vi "Shooter_Begin.vi"   [LabVIEW 2012]
uses:
  <vilib>/Rock Robotics/WPI/CAN/Jaguar/SubVIs/WPI_CANJaguar_ControlMode.ctl
  <vilib>/Rock Robotics/SystemInterfaces/DIO/FPGA_DIOChannel.ctl
  <vilib>/Rock Robotics/SystemInterfaces/Typedef/FPGA_TypedefDigitalModule.ctl
  <vilib>/Rock Robotics/WPI/CAN/Jaguar/SubVIs/WPI_CANJaguar_BrakeCoastMode.ctl
  Program Files (x86)/National Instruments/LabVIEW 2012/examples/FRC/I2C/ADXL345 I2C/Driver/ADXL345 I2C Range.ctl
  <vilib>/Rock Robotics/WPI/MotorControl/WPI_MotorControlOpenCANJaguar.vi
types:
  T1 = typedef "WPI_CANJaguar_BrakeCoastMode.ctl" = enum8{"Jumper", "Brake", "Coast"}
  T2 = typedef "FPGA_TypedefDigitalModule.ctl" = enum16{"Digital Module 1", "Digital Module 2"}
  T3 = typedef "FPGA_DIOChannel.ctl" = enum8{"DIO 1", "DIO 2", "DIO 3", "DIO 4", "DIO 5", "DIO 6", "DIO 7", "DIO 8", "DIO 9", "DIO 10", "DIO 11", "DIO 12", "DIO 13", "DIO 14", "Invalid"}
  T4 = typedef "WPI_CANJaguar_ControlMode.ctl" = enum8{"Percent VBus", "Current", "Speed", "Position", "Voltage"}
  T5 = typedef "WPI_MotorControlDeviceRef.ctl" = cluster{"DeviceStatus":errorcluster, "Type":enum16{"PWM", "CAN"}, "PWM":cluster{"Digital Module":T2, "PWM Channel":T6, "DeadBand":T7}, "CAN":cluster{"Device Number":u8, "Control Mode":T4, "Semaphore":T8, "Max Vout":dbl}, "Invert":bool, "TransformRef":T9, "InvTransformRef":T9}
  T6 = typedef "FPGA_DIOPWMChannel.ctl" = enum8{"PWM 1", "PWM 2", "PWM 3", "PWM 4", "PWM 5", "PWM 6", "PWM 7", "PWM 8", "PWM 9", "PWM 10", "Invalid"}
  T7 = typedef "WPI_PWMDeadband.ctl" = cluster{"Name":string, "maxPositivePwm":i32, "minPositivePwm":i32, "centerPwm":i32, "maxNegativePwm":i32, "minNegativePwm":i32, "angularRange":u16}
  T8 = typedef "Semaphore RefNum" = refnum<k1>
  T9 = typedef "WPI_PWMTransform_ConPane.ctl" = refnum<vi>
  T10 = typedef "ADXL345 I2C Range.ctl" = u8
  T11 = typedef "WPI_I2CDevRef.ctl" = cluster{"DevStatus":errorcluster, "Digital Module":T2, "Device Address":u8}
  T12 = typedef "WPI_DigitalInputDevRef.ctl" = cluster{"DevStatus":errorcluster, "DIO Channel":T3, "Digital Module":T2}
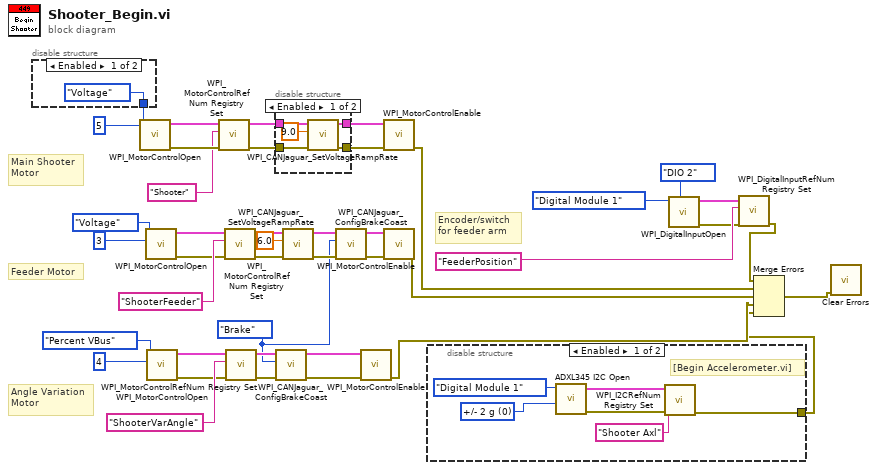
[diagram p0: block diagram]
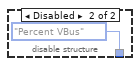
[diagram p4: hidden frame]
diagram:
  w7 = WPI_CANJaguar_BrakeCoastMode."Brake" ("Brake / Coast Mode")
  # "Angle Variation\nMotor"
  # "Main Shooter\nMotor"
  # "Feeder Motor"
  # "Encoder/switch\nfor feeder arm"
  n1 = disable-structure shown="Enabled" {
    disable-tunnel: [WPI_CANJaguar_ControlMode."Voltage" ("Control Mode") WPI_CANJaguar_ControlMode."Percent VBus" ("Control Mode")] -> w31
    frame Enabled {
    }
    frame Disabled {
    }
  }
  n2 = call-poly <vilib>:"WPI_MotorControlOpen.vi"("Device Number"=u8 5, "Control Mode"=w31) -> ("error out"=w34:errorcluster, "MotorControlDeviceRef"=w35:T5)  [unwired: 8 in]
  n3 = call-poly <vilib>:"WPI_MotorControlOpen.vi"("Device Number"=u8 3, "Control Mode"=WPI_CANJaguar_ControlMode."Voltage") -> ("error out"=w38:errorcluster, "MotorControlDeviceRef"=w41:T5)  [unwired: 8 in]
  n4 = call-poly <vilib>:"WPI_MotorControlOpen.vi"("Device Number"=u8 4, "Control Mode"=WPI_CANJaguar_ControlMode."Percent VBus") -> ("error out"=w23:errorcluster, "MotorControlDeviceRef"=w26:T5)  [unwired: 8 in]
  n5 = call <vilib>:"WPI_MotorControlRefNum Registry Set.vi"("error in (no error)"=w34, "refnum name"="Shooter", "MotorControlDevRef"=w35) -> ("error out"=w28:errorcluster, "MotorControlDevRef"=w30:T5)  [unwired: 7 in]
  n6 = call <vilib>:"WPI_MotorControlRefNum Registry Set.vi"("error in (no error)"=w38, "refnum name"="ShooterFeeder", "MotorControlDevRef"=w41) -> ("error out"=w12:errorcluster, "MotorControlDevRef"=w39:T5)  [unwired: 7 in]
  n7 = call <vilib>:"WPI_MotorControlRefNum Registry Set.vi"("error in (no error)"=w23, "refnum name"="ShooterVarAngle", "MotorControlDevRef"=w26) -> ("error out"=w15:errorcluster, "MotorControlDevRef"=w24:T5)  [unwired: 7 in]
  n8 = disable-structure shown="Enabled" {
    disable-tunnel: w30 -> [w49 _]
    disable-tunnel: [w48 _] -> w29
    disable-tunnel: w28 -> [w47 _]
    disable-tunnel: [w46 _] -> w27
    frame Enabled {
      n9 = call <vilib>:"WPI_CANJaguar_SetVoltageRampRate.vi"("error in (no error)"=w47, "VoltageRampRate (V/s)"=9.0, "CAN Jaguar Ref"=w49) -> ("error out"=w46:errorcluster, "CAN Jaguar Ref Out"=w48:T5)  [unwired: 7 in]
    }
    frame Disabled {
    }
  }
  n10 = call <vilib>:"WPI_CANJaguar_ConfigBrakeCoast.vi"("error in (no error)"=w15, "Brake / Coast Mode"=w7, "CAN Jaguar Ref"=w24) -> ("error out"=w14:errorcluster, "CAN Jaguar Ref Out"=w16:T5)  [unwired: 7 in]
  n11 = call <vilib>:"WPI_CANJaguar_SetVoltageRampRate.vi"("error in (no error)"=w12, "VoltageRampRate (V/s)"=6.0, "CAN Jaguar Ref"=w39) -> ("error out"=w9:errorcluster, "CAN Jaguar Ref Out"=w13:T5)  [unwired: 7 in]
  n12 = call <vilib>:"WPI_CANJaguar_ConfigBrakeCoast.vi"("error in (no error)"=w9, "Brake / Coast Mode"=w7, "CAN Jaguar Ref"=w13) -> ("error out"=w8:errorcluster, "CAN Jaguar Ref Out"=w10:T5)  [unwired: 7 in]
  n13 = call <vilib>:"WPI_MotorControlEnable.vi"("error in (no error)"=w14, "CAN Jaguar Ref"=w16) -> ("error out"=w4:errorcluster)  [unwired: 8 in, 1 out]
  n14 = call <vilib>:"WPI_MotorControlEnable.vi"("error in (no error)"=w27, "CAN Jaguar Ref"=w29) -> ("error out"=w6:errorcluster)  [unwired: 8 in, 1 out]
  n15 = call <vilib>:"WPI_MotorControlEnable.vi"("error in (no error)"=w8, "CAN Jaguar Ref"=w10) -> ("error out"=w5:errorcluster)  [unwired: 8 in, 1 out]
  n16 = disable-structure shown="Enabled" {
    disable-tunnel: [w50 _] -> w3
    frame Enabled {
      w54 = T10 0 items=["+/- 2 g", "+/- 4 g", "+/- 8 g", "+/- 16 g"] ("Range")
      # "[Begin Accelerometer.vi]"
      n17 = call "ADXL345 I2C Open.vi"("Range"=w54, "DIO Module (Module 1)"=FPGA_TypedefDigitalModule."Digital Module 1") -> ("error out"=w51:errorcluster, "I2CDevRef"=w53:T11)  [unwired: 8 in]
      n18 = call <vilib>:"WPI_I2CRefNum Registry Set.vi"("error in (no error)"=w51, "refnum name"="Shooter Axl", "I2CDevRef"=w53) -> ("error out"=w50:errorcluster)  [unwired: 7 in, 1 out]
    }
    frame Disabled {
    }
  }
  n19 = call <vilib>:"WPI_DigitalInputOpen.vi"("DIO Channel"=FPGA_DIOChannel."DIO 2", "Digital Module (Module 1)"=FPGA_TypedefDigitalModule."Digital Module 1") -> ("error out"=w19:errorcluster, "DigitalInputDevRef"=w20:T12)  [unwired: 8 in]
  n20 = call <vilib>:"WPI_DigitalInputRefNum Registry Set.vi"("error in (no error)"=w19, "refnum name"="FeederPosition", "DigitalInputDevRef"=w20) -> ("error out"=w2:errorcluster)  [unwired: 7 in, 1 out]
  n21 = Merge Errors(w2, w6, w5, w4, w3) -> (w1:errorcluster)
  n22 = call <vilib>:"Clear Errors.vi"("error in (no error)"=w1) -> ()  [unwired: 6 in, 1 out]
